vi "Vision Processing Glenn.vi"(2 "error in (no error)":errorcluster, 3 "Camera Type":enum16{"206", "1011"}(ring)=enum."1011", 4 "Camera Name":string="Camera") -> (0 "Target Info":T1(array[cluster]))   [LabVIEW 2012]
uses:
  Robot Global Data.vi
  <vilib>/vision/NI_Vision_Development_Module.lvlib
panel:
  in  "Don't loop?":bool
  in  "File Path":path
  in  "Make Target Info":T1(array[cluster])
  in  "Actual process images? (Yes/No)":bool=TRUE
  out "zoomed binary":T2(plugin-control)
  in  "View":bool
  in  "Area Size Limit":i32=444
  in  "Particle Count Limit":i32=8
  in  "Score Limits":T3={"Rect Coverage"=76.0, "Aspect Ratio"=70.0, "X Edge Strength"=40.0, "Y Edge Strength"=60.0}
  in  "Processing":enum32{"Color", "Intensity", "Intensity Open"}(tab)
  in  "Luminance":i32=70
  in  "Saturation":i32=200
  in  "Hue":i32(knob)=118 scale=0.0..255.0
  in  "Margins":cluster{"Hue":i32, "Sat":i32, "Lum":i32}={"Hue"=40, "Sat"=25, "Lum"=25} {"Sat" scale=0.0..40.0; "Lum" scale=0.0..40.0; "Hue" scale=0.0..40.0}
  in  "Range":cluster{"Lower value":sgl, "Upper value":sgl}={"Lower value"=150.0, "Upper value"=255.0} {"Lower value" scale=0.0..255.0; "Upper value" scale=0.0..255.0}
  in  "Range":cluster{"Lower value":sgl, "Upper value":sgl}={"Lower value"=150.0, "Upper value"=255.0} {"Lower value" scale=0.0..255.0; "Upper value" scale=0.0..255.0}
  in  "View":bool
  out "Processed Image":T2(plugin-control)
  out "Original Image":T2(plugin-control)
  # "Instructions:\nProcessing the reflective tape that is illuminated by a ring light can be based\non color or light intensity.\nParticles within the image are scored by rectangle coverage, aspect ratio, and\nfor being hollow with a bold edge. A particle is considered a target if all scores\nare above the score limits. Particles can be annotated -- surrounded by\na rectangle and scores drawn to the left .\nTo control the number of particles being scored, use the count limit and the size\nlimit."
  # "To debug, Enable using the View button.\nFor color processing, you can click in the image to select the color for processing."
  # "Enable by clicking the View button.\nGreen scores are above the limit, orange are below. Inner/outer rect\nindicates all passed."
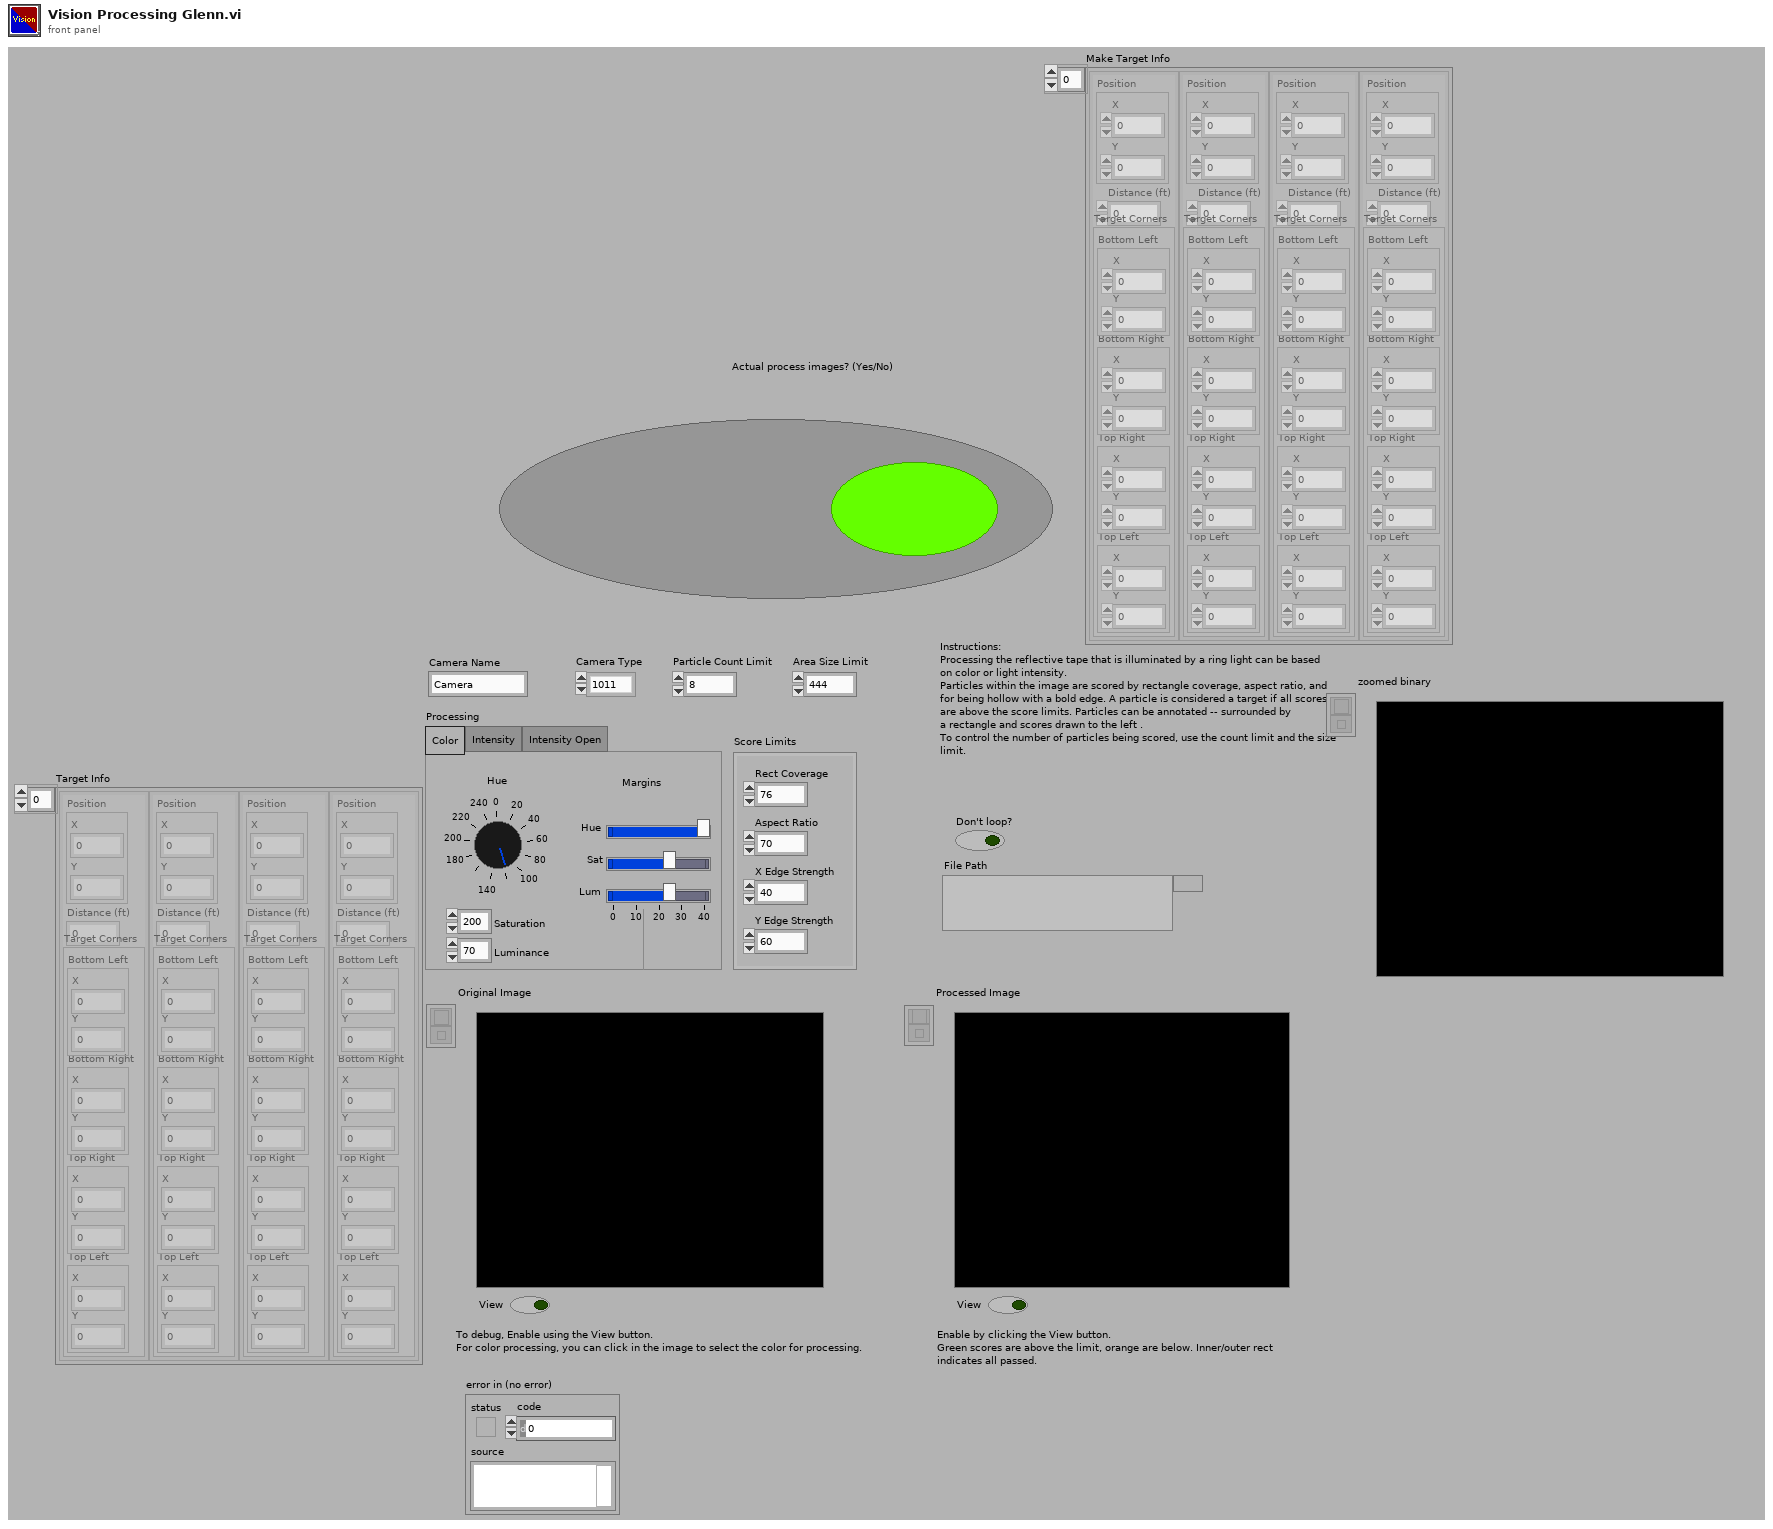
[diagram p1: front panel]
types:
  T1 = cluster{"Position":cluster{"X":dbl, "Y":dbl}, "Distance (ft)":dbl, "Target Corners":cluster{"Bottom Left":cluster{"X":dbl, "Y":dbl}, "Bottom Right":cluster{"X":dbl, "Y":dbl}, "Top Right":cluster{"X":dbl, "Y":dbl}, "Top Left":cluster{"X":dbl, "Y":dbl}}}[]
  T2 = typedef "IMAQ Image.ctl" = refnum<image>
  T3 = cluster{"Rect Coverage":dbl, "Aspect Ratio":dbl, "X Edge Strength":dbl, "Y Edge Strength":dbl}
  T4 = enum32{"AutoM", "Close", "Dilate", "Erode", "Gradient", "Gradient out", "Gradient in", "Hit miss", "Open", "PClose", "POpen", "Thick", "Thin"}
  T5 = typedef "Image Type" = u32
  T6 = typedef "WPI_CameraDevRef.ctl" = cluster{"Camera Address":string, "CameraStatus":errorcluster, "Acquire Image Notifier":refnum<notifier>}
  T7 = typedef "WPI_CameraImageSize.ctl" = enum16{"640x480", "320x240", "160x120"}
  T8 = cluster{cluster{"Left":dbl, "Top":dbl, "Right":dbl, "Bottom":dbl}, dbl[], "Target Corners":cluster{"Bottom Left":cluster{"X":dbl, "Y":dbl}, "Bottom Right":cluster{"X":dbl, "Y":dbl}, "Top Right":cluster{"X":dbl, "Y":dbl}, "Top Left":cluster{"X":dbl, "Y":dbl}}}[]
  T9 = cluster{"Bottom Left":cluster{"X":dbl, "Y":dbl}, "Bottom Right":cluster{"X":dbl, "Y":dbl}, "Top Right":cluster{"X":dbl, "Y":dbl}, "Top Left":cluster{"X":dbl, "Y":dbl}}
  T10 = cluster{"Target Center (-1 to 1)":cluster{"X":dbl, "Y":dbl}, "Distance (ft)":dbl, "Target Corners":cluster{"Bottom Left":cluster{"X":dbl, "Y":dbl}, "Bottom Right":cluster{"X":dbl, "Y":dbl}, "Top Right":cluster{"X":dbl, "Y":dbl}, "Top Left":cluster{"X":dbl, "Y":dbl}}}
  T11 = cluster{"Target Center (-1 to 1)":cluster{"X":dbl, "Y":dbl}, "Distance (ft)":dbl, "Target Corners":cluster{"Bottom Left":cluster{"X":dbl, "Y":dbl}, "Bottom Right":cluster{"X":dbl, "Y":dbl}, "Top Right":cluster{"X":dbl, "Y":dbl}, "Top Left":cluster{"X":dbl, "Y":dbl}}}[]
  T12 = cluster{"Scored Particle Info[0]":cluster{cluster{"Left":dbl, "Top":dbl, "Right":dbl, "Bottom":dbl}, dbl[], "Target Corners":cluster{"Bottom Left":cluster{"X":dbl, "Y":dbl}, "Bottom Right":cluster{"X":dbl, "Y":dbl}, "Top Right":cluster{"X":dbl, "Y":dbl}, "Top Left":cluster{"X":dbl, "Y":dbl}}}, "Scored Particle Info[1]":cluster{cluster{"Left":dbl, "Top":dbl, "Right":dbl, "Bottom":dbl}, dbl[], "Target Corners":cluster{"Bottom Left":cluster{"X":dbl, "Y":dbl}, "Bottom Right":cluster{"X":dbl, "Y":dbl}, "Top Right":cluster{"X":dbl, "Y":dbl}, "Top Left":cluster{"X":dbl, "Y":dbl}}}, "Scored Particle Info[2]":cluster{cluster{"Left":dbl, "Top":dbl, "Right":dbl, "Bottom":dbl}, dbl[], "Target Corners":cluster{"Bottom Left":cluster{"X":dbl, "Y":dbl}, "Bottom Right":cluster{"X":dbl, "Y":dbl}, "Top Right":cluster{"X":dbl, "Y":dbl}, "Top Left":cluster{"X":dbl, "Y":dbl}}}, "Scored Particle Info[3]":cluster{cluster{"Left":dbl, "Top":dbl, "Right":dbl, "Bottom":dbl}, dbl[], "Target Corners":cluster{"Bottom Left":cluster{"X":dbl, "Y":dbl}, "Bottom Right":cluster{"X":dbl, "Y":dbl}, "Top Right":cluster{"X":dbl, "Y":dbl}, "Top Left":cluster{"X":dbl, "Y":dbl}}}, "Scored Particle Info[4]":cluster{cluster{"Left":dbl, "Top":dbl, "Right":dbl, "Bottom":dbl}, dbl[], "Target Corners":cluster{"Bottom Left":cluster{"X":dbl, "Y":dbl}, "Bottom Right":cluster{"X":dbl, "Y":dbl}, "Top Right":cluster{"X":dbl, "Y":dbl}, "Top Left":cluster{"X":dbl, "Y":dbl}}}, "Scored Particle Info[5]":cluster{cluster{"Left":dbl, "Top":dbl, "Right":dbl, "Bottom":dbl}, dbl[], "Target Corners":cluster{"Bottom Left":cluster{"X":dbl, "Y":dbl}, "Bottom Right":cluster{"X":dbl, "Y":dbl}, "Top Right":cluster{"X":dbl, "Y":dbl}, "Top Left":cluster{"X":dbl, "Y":dbl}}}, "Scored Particle Info[6]":cluster{cluster{"Left":dbl, "Top":dbl, "Right":dbl, "Bottom":dbl}, dbl[], "Target Corners":cluster{"Bottom Left":cluster{"X":dbl, "Y":dbl}, "Bottom Right":cluster{"X":dbl, "Y":dbl}, "Top Right":cluster{"X":dbl, "Y":dbl}, "Top Left":cluster{"X":dbl, "Y":dbl}}}, "Scored Particle Info[7]":cluster{cluster{"Left":dbl, "Top":dbl, "Right":dbl, "Bottom":dbl}, dbl[], "Target Corners":cluster{"Bottom Left":cluster{"X":dbl, "Y":dbl}, "Bottom Right":cluster{"X":dbl, "Y":dbl}, "Top Right":cluster{"X":dbl, "Y":dbl}, "Top Left":cluster{"X":dbl, "Y":dbl}}}, "Scored Particle Info[8]":cluster{cluster{"Left":dbl, "Top":dbl, "Right":dbl, "Bottom":dbl}, dbl[], "Target Corners":cluster{"Bottom Left":cluster{"X":dbl, "Y":dbl}, "Bottom Right":cluster{"X":dbl, "Y":dbl}, "Top Right":cluster{"X":dbl, "Y":dbl}, "Top Left":cluster{"X":dbl, "Y":dbl}}}}
  T13 = cluster{"Left":dbl, "Top":dbl, "Right":dbl, "Bottom":dbl}
  T14 = cluster{cluster{"Left":dbl, "Top":dbl, "Right":dbl, "Bottom":dbl}, dbl[], "Target Corners":cluster{"Bottom Left":cluster{"X":dbl, "Y":dbl}, "Bottom Right":cluster{"X":dbl, "Y":dbl}, "Top Right":cluster{"X":dbl, "Y":dbl}, "Top Left":cluster{"X":dbl, "Y":dbl}}}
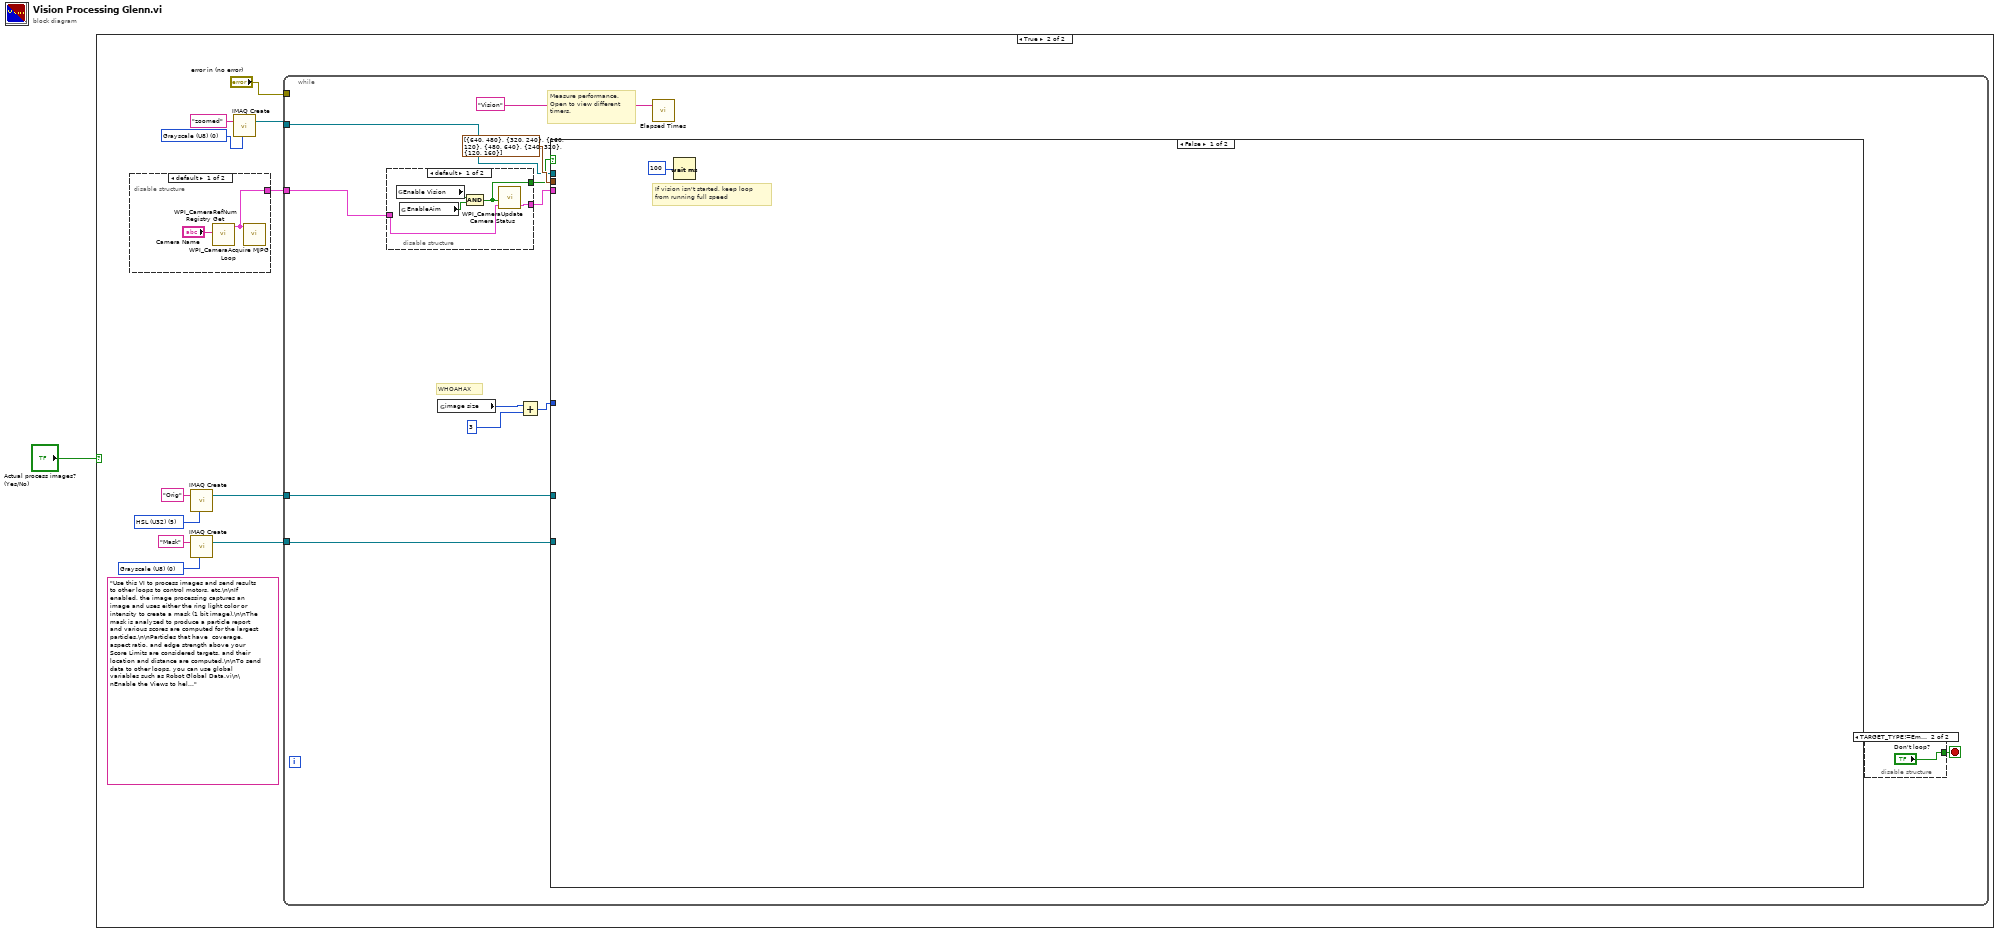
[diagram p0: block diagram]
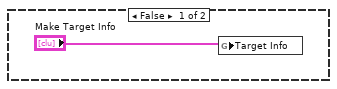
[diagram p2: hidden frame]
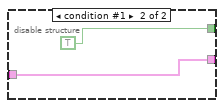
[diagram p4: hidden frame]
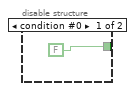
[diagram p5: hidden frame]
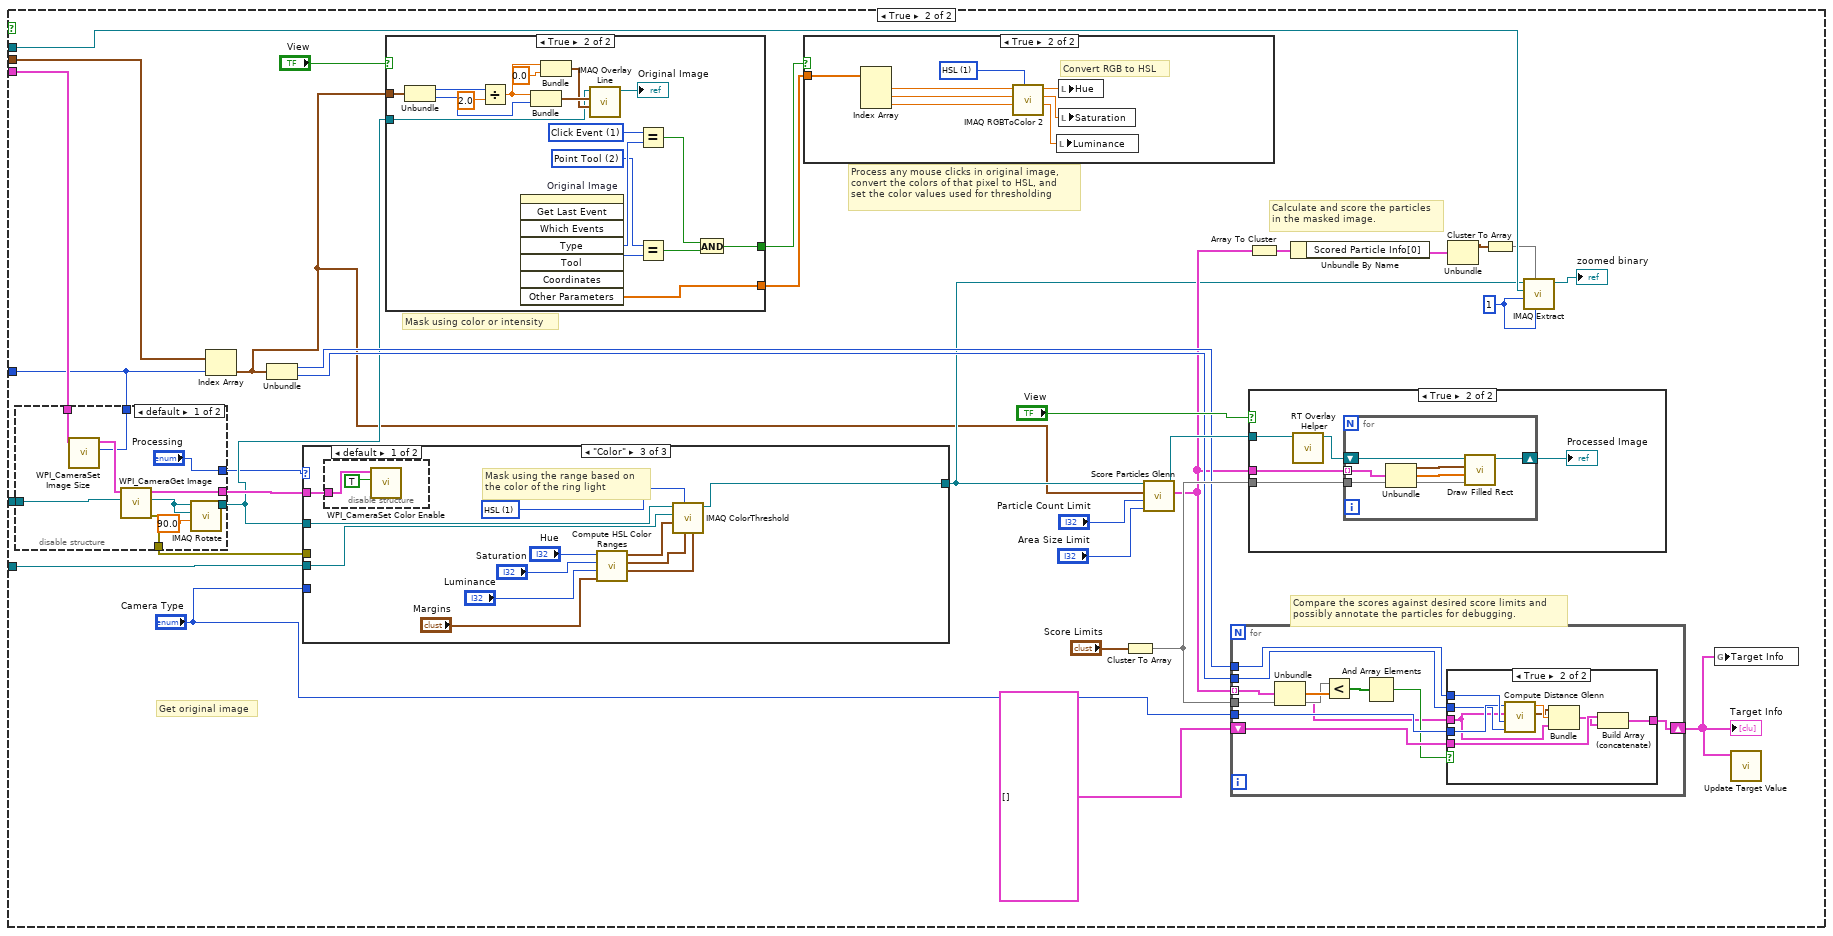
[diagram p6: hidden frame]
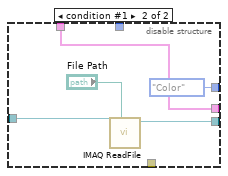
[diagram p7: hidden frame]
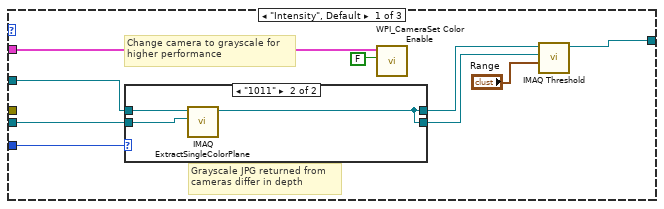
[diagram p9: hidden frame]
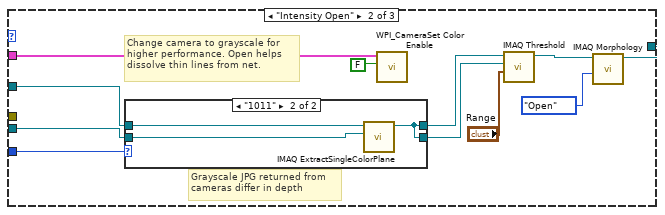
[diagram p11: hidden frame]
diagram:
  n1 = case shown="True" "Actual process images? (Yes/No)" {
    frame False {
      n2 = global write "Robot Global Data.vi" "Target Info"("Make Target Info") -> ()
    }
    frame True {
      w4 = T5 0 items=["Grayscale (U8)", "Grayscale (I16)", "Grayscale (SGL)", "Complex (CSG)", "RGB (U32)", "HSL (U32)", "RGB (U64)", "Grayscale (U16)"] ("Image Type")
      w8 = T5 0 items=["Grayscale (U8)", "Grayscale (I16)", "Grayscale (SGL)", "Complex (CSG)", "RGB (U32)", "HSL (U32)", "RGB (U64)", "Grayscale (U16)"] ("Image Type")
      (unwired) "Use this VI to process images and send results to other loops to control motors, etc.\n\nIf enabled, the image processing captures an image and uses either the ring light color or intensity to create a mask (1 bit image).\n\nThe mask is analyzed to produce a particle report and various scores are computed for the largest particles.\n\nParticles that have  coverage, aspect ratio, and edge strength above your Score Limits are considered targets, and their location and distance are computed.\n\nTo send data to other loops, you can use global variables such as Robot Global Data.vi\n\nEnable the Views to help debug color settings. Disable the View to speed up processing."
      w12 = T5 5 items=["Grayscale (U8)", "Grayscale (I16)", "Grayscale (SGL)", "Complex (CSG)", "RGB (U32)", "HSL (U32)", "RGB (U64)", "Grayscale (U16)"] ("Image Type")
      n3 = disable-structure shown="default" {
        disable-tunnel: [w14 _] -> w10
        frame condition #0 (active) {
          n4 = call <vilib>:"WPI_CameraRefNum Registry Get.vi"("refnum name"="Camera Name") -> ("CameraDevRef"=w14:T6)  [unwired: 9 in, 1 out]
          n5 = call <vilib>:"WPI_CameraAcquire MJPG Loop.vi"("CameraDevRef"=w14) -> ()  [unwired: 11 in]
        }
        frame condition #1 {
        }
      }
      n6 = call "IMAQ Create"("Image Name"="Orig", "Image Type"=w12) -> ("New Image"=w11:T2)  [unwired: 2 in, 2 out]
      n7 = call "IMAQ Create"("Image Name"="Mask", "Image Type"=w8) -> ("New Image"=w6:T2)  [unwired: 2 in, 2 out]
      n8 = call "IMAQ Create"("Image Name"="zoomed", "Image Type"=w4) -> ("New Image"=w3:T2)  [unwired: 2 in, 2 out]
      n9 = while {
        tunnel: w11 -> [w26]
        tunnel: w10 -> [w25]
        tunnel: "error in (no error)" -> [_]
        tunnel: w6 -> [w22]
        tunnel: w3 -> [w20]
        stop <- w27 stop-if-true
        # "WHOAHAX"
        # "Measure performance.\nOpen to view different\ntimers."
        n10 = disable-structure shown="default" {
          disable-tunnel: w25 -> [w32 w34]
          disable-tunnel: [w31 w34] -> w24
          disable-tunnel: [w28 TRUE] -> w19
          frame condition #0 (active) {
            n11 = global read "Robot Global Data.vi" "Enable Vision"() -> (w30:bool)
            n12 = global read "Robot Global Data.vi" "EnableAim"() -> (w29:bool)
            n13 = And(x=w30, y=w29) -> (x .and. y?=w28:bool)
            n14 = call <vilib>:"WPI_CameraUpdate Camera Status.vi"("CameraDevRef In"=w32, "Enable Vision"=w28) -> ("CameraDevRef Out"=w31:T6)  [unwired: 3 in]
          }
          frame condition #1 {
          }
        }
        n15 = global read "Robot Global Data.vi" "image size"() -> (w18:T7)
        n16 = Add(x=w18, y=3) -> (x+y=w16:i32)
        n17 = case shown="False" w19 {
          tunnel: w26 -> [_ w50]
          tunnel: w24 -> [_ w61]
          tunnel: w16 -> [_ w57]
          tunnel: w22 -> [_ w53]
          tunnel: cluster{i32, i32}[] [{640, 480}, {320, 240}, {160, 120}, {480, 640}, {240, 320}, {120, 160}] -> [_ w56]
          tunnel: w20 -> [_ w51]
          frame False {
            # "If vision isn't started, keep loop\nfrom running full speed"
            n18 = Wait (ms)(milliseconds to wait=u32 100) -> ()  [unwired: 1 out]
          }
          frame True {
            w44 = 1 ("X Step Size")
            # "Compare the scores against desired score limits and\npossibly annotate the particles for debugging."
            # "Process any mouse clicks in original image,\nconvert the colors of that pixel to HSL, and\nset the color values used for thresholding"
            # "Calculate and score the particles\nin the masked image."
            # "Mask using color or intensity"
            # "Get original image"
            n19 = disable-structure shown="default" {
              disable-tunnel: [w80 w85] -> w63
              disable-tunnel: [w79 _] -> w62
              disable-tunnel: w61 -> [w77 w85]
              disable-tunnel: w57 -> [w76 _]
              disable-tunnel: w50 -> [w75 w83]
              disable-tunnel: [w72 w82] -> w40
              disable-tunnel: ["Processing" enum32{"Color", "Intensity", "Intensity Open"}."Color" ("Processing")] -> w39
              frame condition #0 (active) {
                n20 = call <vilib>:"WPI_CameraSet Image Size.vi"("Image Size"=w76, "CameraDevRef"=w77) -> ("CameraDevRef Out"=w78:T6)  [unwired: 8 in, 1 out]
                n21 = call <vilib>:"WPI_CameraGet Image.vi"("Image"=w75, "CameraDevRef"=w78) -> ("error out"=w79:errorcluster, "Image Out"=w74:T2, "CameraDevRef Out"=w80:T6)  [unwired: 7 in]
                n22 = call "IMAQ Rotate"("Angle (degrees)"=sgl 90.0, "Image Dst"=w74, "Image Src"=w74) -> ("Image Dst Out"=w72:T2)  [unwired: 7 in, 1 out]
              }
              frame condition #1 {
                n23 = call "IMAQ ReadFile"("File Path"="File Path", "Image"=w83) -> ("Image Out"=w82:T2)  [unwired: 5 in, 4 out]
              }
            }
            n24 = Index Array(array=w56, index=w57) -> (element=w38:cluster{i32, i32})
            n25 = Unbundle(w38) -> (w55:i32, w54:i32)
            n26 = case shown="\"Color\"" w39 {
              tunnel: w40 -> [w98 w110 w135]
              tunnel: [w101 w115 w134] -> w46
              tunnel: w63 -> [w99 w113 w125]
              tunnel: w62 -> [_ _ _]
              tunnel: w53 -> [w97 w111 w124]
              tunnel: "Camera Type" -> [w96 w112 _]
              frame "Intensity", Default {
                # "Grayscale JPG returned from\ncameras differ in depth"
                # "Change camera to grayscale for\nhigher performance"
                n27 = case shown="\"1011\"" w96 {
                  tunnel: w98 -> [w104 w107]
                  tunnel: w97 -> [w103 w106]
                  tunnel: [w104 w105] -> w95
                  tunnel: [w103 w105] -> w94
                  frame "206", Default {
                  }
                  frame "1011" {
                    n28 = call "IMAQ ExtractSingleColorPlane"("Image Dst"=w106, "Image Src"=w107) -> ("Image Dst Out"=w105:T2)  [unwired: 8 in, 1 out]
                  }
                }
                n29 = call <vilib>:"WPI_CameraSet Color Enable.vi"("Color Enabled"=FALSE, "CameraDevRef"=w99) -> ()  [unwired: 8 in, 2 out]
                n30 = call "IMAQ Threshold"("Range"="Range", "Image Dst"=w94, "Image Src"=w95) -> ("Image Dst Out"=w101:T2)  [unwired: 3 in, 5 out]
              }
              frame "Intensity Open" {
                # "Grayscale JPG returned from\ncameras differ in depth"
                # "Change camera to grayscale for\nhigher performance. Open helps\ndissolve thin lines from net."
                n31 = case shown="\"1011\"" w112 {
                  tunnel: w110 -> [w120 w123]
                  tunnel: w111 -> [w119 w122]
                  tunnel: [w120 w121] -> w109
                  tunnel: [w119 w121] -> w108
                  frame "206", Default {
                  }
                  frame "1011" {
                    n32 = call "IMAQ ExtractSingleColorPlane"("Image Dst"=w122, "Image Src"=w123) -> ("Image Dst Out"=w121:T2)  [unwired: 8 in, 1 out]
                  }
                }
                n33 = call <vilib>:"WPI_CameraSet Color Enable.vi"("Color Enabled"=FALSE, "CameraDevRef"=w113) -> ()  [unwired: 8 in, 2 out]
                n34 = call "IMAQ Threshold"("Range"="Range", "Image Dst"=w108, "Image Src"=w109) -> ("Image Dst Out"=w116:T2)  [unwired: 3 in, 5 out]
                n35 = call "IMAQ Morphology"("Operation"=T4."Open", "Image Src"=w116) -> ("Image Dst Out"=w115:T2)  [unwired: 8 in, 1 out]
              }
              frame "Color" {
                w133 = u16 1 items=["RGB", "HSL", "HSV", "HSI"] ("Color Mode")
                # "Mask using the range based on\nthe color of the ring light"
                n36 = disable-structure shown="default" {
                  disable-tunnel: w125 -> [w137 _]
                  frame condition #0 (active) {
                    n37 = call <vilib>:"WPI_CameraSet Color Enable.vi"("Color Enabled"=TRUE, "CameraDevRef"=w137) -> ()  [unwired: 8 in, 2 out]
                  }
                  frame condition #1 {
                  }
                }
                n38 = call "Compute HSL Color Ranges.vi"("Margins"="Margins", "Luminance"="Luminance", "Saturation"="Saturation", "Hue"="Hue") -> ("Lum Range"=w130:cluster{i32, i32}, "Sat Range"=w131:cluster{i32, i32}, "Hue Range"=w132:cluster{i32, i32})  [unwired: 5 in]
                n39 = call "IMAQ ColorThreshold"("Blue or Luma or Val or Inten Range"=w130, "Green or Sat Range"=w131, "Color Mode"=w133, "Red or Hue Range"=w132, "Image Dst"=w124, "Image Src"=w135) -> ("Image Dst Out"=w134:T2)  [unwired: 4 in, 1 out]
              }
            }
            n40 = case shown="True" "View" {
              tunnel: w40 -> [_ w151]
              tunnel: [_ w162] -> w59
              tunnel: [_ w159] -> w58
              tunnel: w38 -> [_ w150]
              frame False {
              }
              frame True {
                w160 = 2 items=["None", "Selection Tool", "Point Tool", "Line Tool", "Rectangle Tool", "Oval Tool", "Polygon Tool", "ClosedFreehandTool", "Annulus Tool", "Rotated Rectangle Tool", "Zoom Tool", "Pan Tool", "Polyline Tool", "Freehand Tool"] ("Tool")
                w161 = 1 items=["No Event"=0, "Click Event"=1, "Draw Event"=2, "Size Event"=4, "Scroll Event"=5, "Double Click Event"=8] ("Type")
                n41 = Unbundle(w150) -> (w154:i32, w153:i32)
                n42 = Divide(x=w154, y=2.0) -> (x/y=w152:dbl)
                n43 = invoke on="Original Image" class="ImageControl" method="Get Last Event"() -> ("Type"=w163:i32, "Tool"=w166:i32, "Other Parameters"=w159:sgl[])  [unwired: 8 in, 5 out]
                n44 = Bundle(w152, w153) -> (w157:cluster{dbl, i32})  [unwired: 1 in]
                n45 = Bundle(w152, "element"=0.0) -> (w155:cluster{dbl, "element":dbl})  [unwired: 1 in]
                n46 = call "IMAQ Overlay Line"("End Point"=w155, "Start Point"=w157, "Image"=w151) -> ("Image Out"=→"Original Image":T2)  [unwired: 7 in, 1 out]
                n47 = Equal?(x=w161, y=w163) -> (x = y?=w164:bool)
                n48 = Equal?(x=w160, y=w166) -> (x = y?=w165:bool)
                n49 = And(x=w164, y=w165) -> (x .and. y?=w162:bool)
              }
            }
            n50 = case shown="True" w59 {
              tunnel: w58 -> [_ w93]
              frame False {
              }
              frame True {
                w92 = u16 1 items=["RGB", "HSL", "HSV", "HSI", "CIE L*a*b*", "CIE XYZ"] ("Color Mode")
                # "Convert RGB to HSL"
                n51 = Index Array(array=w93) -> (element #1=w91:sgl, element #2=w89:sgl, element #3=w87:sgl)  [unwired: 3 in]
                n52 = call "IMAQ RGBToColor 2"("Color Mode"=w92, "Blue value"=w87, "Green value"=w89, "Red value"=w91) -> ("Blue or Luma or Val or Inten or Z or b*value"=w86:dbl, "Green or Sat or Y or a* value"=w88:dbl, "Red or Hue or X or L* value"=w90:dbl)  [unwired: 4 in, 1 out]
                n53 = local write "Luminance"(w86) -> ()
                n54 = local write "Hue"(w90) -> ()
                n55 = local write "Saturation"(w88) -> ()
              }
            }
            n56 = Cluster To Array(cluster="Score Limits") -> (array=w66:dbl[])
            n57 = call "Score Particles Glenn.vi"("Area Size Limit"="Area Size Limit", "Particle Count Limit"="Particle Count Limit", "Dimensions"=w38, "Image Refnum in"=w46) -> ("Scored Particle Info"=w49:T8, "Image Refnum out"=w70:T2)  [unwired: 6 in]
            n58 = for {
              shift-right: [w176] -> w41
              shift-left: T1 [] -> [w177]
              tunnel: w55 -> [w175]
              tunnel: w49 -> [w174] mode=indexing
              tunnel: w66 -> [w169]
              tunnel: "Camera Type" -> [w173]
              tunnel: w54 -> [w168]
              n59 = Unbundle(w174) -> (w170:dbl[], "Target Corners"=w167:T9)  [unwired: 1 out]
              n60 = Less?(x=w169, y=w170) -> (x < y?=w172:bool[])
              n61 = And Array Elements(Boolean array=w172) -> (logical AND=w171:bool)
              n62 = case shown="True" w171 {
                tunnel: w177 -> [w178 w187]
                tunnel: [w178 w186] -> w176
                tunnel: w175 -> [_ w185]
                tunnel: w173 -> [_ w183]
                tunnel: w168 -> [_ w182]
                tunnel: w167 -> [_ w179]
                frame False {
                }
                frame True {
                  n63 = call "Compute Distance Glenn.vi"("Y Image Resolution"=w182, "X Image Resolution"=w185, "Target Corners"=w179, "Camera Type"=w183) -> ("Target Center (-1 to 1)"=w181:cluster{"X":dbl, "Y":dbl}, "Distance (ft)"=w184:dbl)  [unwired: 6 in]
                  n64 = Bundle("Target Center (-1 to 1)"=w181, "Distance (ft)"=w184, "Target Corners"=w179) -> (w180:T10)  [unwired: 1 in]
                  n65 = Build Array (concatenate)(w187, w180) -> (w186:T11)
                }
              }
            }
            "Target Info" <- w41
            n66 = Array To Cluster(array=w49) -> (cluster=w43:T12)
            n67 = case shown="True" "View" {
              tunnel: w70 -> [_ w139]
              tunnel: w49 -> [_ w141]
              tunnel: w66 -> [_ w140]
              frame False {
              }
              frame True {
                n68 = call "RT Overlay Helper.vi"("Refnum in"=w139) -> ("Refnum out"=w142:T2)  [unwired: 10 in]
                n69 = for {
                  shift-right: [w147] -> w138
                  shift-left: w142 -> [w148]
                  tunnel: w141 -> [w144] mode=indexing
                  tunnel: w140 -> [w143]
                  n70 = Unbundle(w144) -> (w145:T13, w146:dbl[])  [unwired: 1 out]
                  n71 = call "Draw Filled Rect.vi"("Limits"=w143, "Scores"=w146, "Bounding Box"=w145, "image in"=w148) -> ("image out"=w147:T2)  [unwired: 7 in]
                }
                "Processed Image" <- w138
              }
            }
            n72 = Unbundle By Name(w43) -> ("Scored Particle Info[0]"=w42:T14)
            n73 = Unbundle(w42) -> (w48:T13)  [unwired: 2 out]
            n74 = Cluster To Array(cluster=w48) -> (array=w47:dbl[])
            n75 = call "IMAQ Extract"("Y Step Size"=w44, "Optional Rectangle"=w47, "X Step Size"=w44, "Image Dst"=w51, "Image Src"=w46) -> ("Image Dst Out"=→"zoomed binary":T2)  [unwired: 5 in, 1 out]
            n76 = global write "Robot Global Data.vi" "Target Info"(w41) -> ()
            n77 = call "Update Target Value.vi"("Target Info"=w41) -> ()  [unwired: 10 in, 1 out]
          }
        }
        n78 = call "Elapsed Times.vi"("Call Name"="Vision") -> ()  [unwired: 2 in, 1 out]
        n79 = disable-structure shown="TARGET_TYPE!=Embedded" {
          disable-tunnel: [FALSE "Don't loop?"] -> w27
          frame condition #0 {
          }
          frame condition #1 (active) {
          }
        }
      }
    }
  }
